vi "fg_path.vi"(8 "error in (no error)":errorcluster, 11 "custom_path":path) -> (0 "error out":errorcluster, 3 "config_working":path)   [LabVIEW 2015, in "lv-build.lvlib"]
doc: "Returns the location for the configuration, if provided a custom path, it will pass that path through."
uses:
  lv-build.lvlib
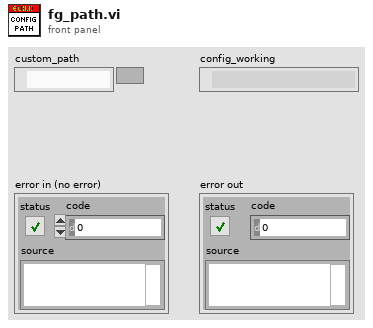
[diagram p1: front panel]
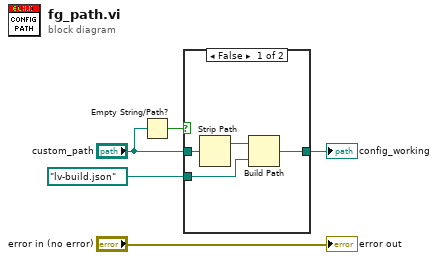
[diagram p0: block diagram]
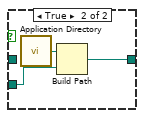
[diagram p2: hidden frame]
diagram:
  n1 = Empty String/Path?(string/path="custom_path") -> (empty?=w5:bool)
  n2 = case shown="False" w5 {
    tunnel: [w7 w12] -> w3
    tunnel: "custom_path" -> [w9 _]
    tunnel: path "lv-build.json" ("Application Directory") -> [w6 w10]
    frame False {
      n3 = Strip Path(path=w9) -> (stripped path=w8:path)  [unwired: 1 out]
      n4 = Build Path(base path=w8, name or relative path=w6) -> (appended path=w7:path)
    }
    frame True {
      n5 = call <vilib>:"Application Directory.vi"() -> ("Application Directory"=w11:path)
      n6 = Build Path(base path=w11, name or relative path=w10) -> (appended path=w12:path)
    }
  }
  "config_working" <- w3
  "error out" <- "error in (no error)"
